vi "New Project.vi"(9 "DBSet":T1={"Server"="172.20.23.107", "DB"="HTPSDB", "PSW"="data'songyy", "User"="sa"}, 10 "UserID":string="L043460", 11 "厂区":string="清溪") -> ()   [LabVIEW 2011] (continued)
                            n505 = Index Array(array=w581) -> (element=w578:bool)  [unwired: 1 in]
                            n506 = local write "fre-save"(w574) -> ()
                            n507 = local write "AutoSN"(w578) -> ()
                          }
                          frame #2 {
                            n508 = disable-structure shown="禁用" {
                              disable-tunnel: w584 -> [w585 _]
                              frame Disabled {
                                n509 = local read "Luxshare_P/N:"() -> (w624:string)
                                n510 = local read "Luxshare_P/N:"() -> (w627:string)
                                n511 = local read "Luxshare_P/N:"() -> (w630:string)
                                n512 = local read "厂区"() -> ()  [unwired: 1 out]
                                n513 = local read "厂区"() -> (w586:string)
                                n514 = call "query.net.vi"() -> ()  [unwired: 10 in, 2 out]
                                n515 = call "_wmg_PNtoPNwhereConnect.vi"("Input"=w624) -> ("Output"=w598:string)
                                n516 = call "_wmg_PNtoPNwhereConnect.vi"("Input"=w630) -> ("Output"=w603:string)
                                n517 = call "_wmg_PNtoPNwhereConnect.vi"("Input"=w627) -> ("Output"=w601:string)
                                n518 = property on="System_Mode" class="Ring (严格)"() -> ("RingText.Text"=w597:string)  [unwired: 2 in, 2 out]
                                n519 = call "_wmg_HardModetoHardModewhereConnect.vi"("Input"=w597, "Factory"=w586) -> ("Output"=w588:string)
                                n520 = Concatenate Strings(w603, w588) -> (w602:string)
                                n521 = call "sql-readinfo_vproject.vi"("DBSet"=w585, "操作模式"=T7."查询数据", "查询项目"="Prjinf", "限定条件"=w602) -> ("ResultString"=w617:string)  [unwired: 13 in, 10 out]
                                n522 = local write "Project Information"(w617) -> ()
                                n523 = Concatenate Strings(w598, w588) -> (w596:string)
                                n524 = call "sql-readinfo_vproject.vi"("DBSet"=w585, "操作模式"=T7."查询数据", "查询项目"="SwitchMatrix", "限定条件"=w596) -> ("ResultString"=w619:string)  [unwired: 13 in, 10 out]
                                n525 = Concatenate Strings(w601, w588) -> (w600:string)
                                n526 = call "sql-readinfo_vproject.vi"("DBSet"=w585, "操作模式"=T7."查询数据", "查询项目"="Spec", "限定条件"=w600) -> ("ResultString"=→"Spec_midVar":string)  [unwired: 13 in, 10 out]
                                n527 = local write "Switch Matrix"(w619) -> ()
                                n528 = local read "Luxshare_P/N:"() -> (w609:string)
                                n529 = local read "Luxshare_P/N:"() -> (w612:string)
                                n530 = local read "Luxshare_P/N:"() -> (w615:string)
                                n531 = local read "Luxshare_P/N:"() -> (w621:string)
                                n532 = call "_wmg_PNtoPNwhereConnect.vi"("Input"=w609) -> ("Output"=w589:string)
                                n533 = Concatenate Strings(w589, w588) -> (w587:string)
                                n534 = call "_wmg_PNtoPNwhereConnect.vi"("Input"=w612) -> ("Output"=w591:string)
                                n535 = Concatenate Strings(w591, w588) -> (w590:string)
                                n536 = call "_wmg_PNtoPNwhereConnect.vi"("Input"=w615) -> ("Output"=w593:string)
                                n537 = Concatenate Strings(w593, w588) -> (w592:string)
                                n538 = call "sql-readinfo_vproject.vi"("DBSet"=w585, "操作模式"=T7."查询数据", "查询项目"="Spec_Points", "限定条件"=w587) -> ("ResultString"=w605:string)  [unwired: 13 in, 10 out]
                                n539 = call "sql-readinfo_vproject.vi"("DBSet"=w585, "操作模式"=T7."查询数据", "查询项目"="Switch_File_Path", "限定条件"=w592) -> ("ResultString"=w607:string)  [unwired: 13 in, 10 out]
                                n540 = call "_wmg_PNtoPNwhereConnect.vi"("Input"=w621) -> ("Output"=w595:string)
                                n541 = Concatenate Strings(w595, w588) -> (w594:string)
                                n542 = call "sql-readinfo_vproject.vi"("DBSet"=w585, "操作模式"=T7."查询数据", "查询项目"="LabelC", "限定条件"=w594) -> ("ResultString"=w618:string)  [unwired: 13 in, 10 out]
                                n543 = call "sql-readinfo_vproject.vi"("DBSet"=w585, "操作模式"=T7."查询数据", "查询项目"="Spec_File_Path", "限定条件"=w590) -> ("ResultString"=w606:string)  [unwired: 13 in, 10 out]
                                n544 = local write "Switch File Path"(w607) -> ()
                                n545 = Decimal String To Number(string=w605) -> (number=w604:i32)  [unwired: 2 in, 1 out]
                                n546 = local write "Spec Points"(w604) -> ()
                                n547 = local write "Spec File Path"(w606) -> ()
                                n548 = local write "Label Content"(w618) -> ()
                              }
                              frame Enabled {
                              }
                            }
                          }
                          frame #3 {
                            n549 = local read "Luxshare_P/N:"() -> (w647:string)
                            n550 = property on="System_Mode" class="Ring (严格)"() -> ("RingText.Text"=w646:string)  [unwired: 2 in, 2 out]
                            n551 = local read "厂区"() -> (w645:string)
                            n552 = Search and Replace String(input string="select SwitchMatrix ,Prjinf,Spec,LabelC,Switch_File_Path,Spec_File_Path,Spec_Points from vproject where LuxsharePN='@PN@' and HardWare_Mode='@Mode@' and  Factory ='@Facotry@'", search string="@PN@" ("搜索字符串"), replace string=w647) -> (result string=w651:string)  [unwired: 5 in, 3 out]
                            n553 = Search and Replace String(input string=w651, search string="@Mode@" ("搜索字符串"), replace string=w646) -> (result string=w649:string)  [unwired: 5 in, 3 out]
                            n554 = Search and Replace String(input string=w649, search string="@Facotry@" ("搜索字符串"), replace string=w645) -> (result string=w644:string)  [unwired: 5 in, 3 out]
                            n555 = call "query.net.vi"("Sql"=w644, "DBSet"=w643) -> ("result"=w642:string[][])  [unwired: 8 in, 1 out]
                            n556 = Index Array(array=w642, index (row)=0 ("索引 (行)")) -> (element=w640:string[])  [unwired: 1 in]
                            n557 = Index Array(array=w640) -> (element #1=w639:string, element #2=w638:string, element #3=w637:string, element #4=w636:string, element #5=w635:string, element #6=w634:string, element #7=w633:string)  [unwired: 7 in]
                            n558 = Decimal String To Number(string=w633) -> (number=w632:i32)  [unwired: 2 in, 1 out]
                            n559 = local write "Switch Matrix"(w639) -> ()
                            n560 = local write "Project Information"(w638) -> ()
                            n561 = local write "Switch File Path"(w635) -> ()
                            n562 = local write "Label Content"(w636) -> ()
                            n563 = local write "Spec_midVar"(w637) -> ()
                            n564 = local write "Spec File Path"(w634) -> ()
                            n565 = local write "Spec Points"(w632) -> ()
                          }
                          frame #4 {
                            n566 = local read "Spec_midVar"() -> (w655:string)
                            n567 = property on="Cable AWG:" class="Ring (严格)"() -> ("StringsAndValues[]"=w666:T10)  [unwired: 2 in, 2 out]
                            n568 = property on="Customer" class="Ring (严格)"() -> ("StringsAndValues[]"=w668:T10)  [unwired: 2 in, 2 out]
                            n569 = Search and Replace String(replace all?=TRUE ("替换全部？(F)"), input string=w655, search string="#" ("搜索字符串"), replace string="\t") -> (result string=w659:string)  [unwired: 4 in, 3 out]
                            n570 = local read "Customer"() -> (w667:string)
                            n571 = local read "AWG"() -> (w665:string)
                            n572 = Spreadsheet String To Array(format string="%s" ("格式字符串"), spreadsheet string=w659, array type (2D Dbl)=string[][] []) -> (array=w654:string[][])  [unwired: 1 in]
                            n573 = call "_wmg_downlistValue.vi"(1:"Customer"=w665, 2:"Customer"=w666) -> ("Customer"=w669:u16)
                            n574 = call "_wmg_downlistValue.vi"(1:"Customer"=w667, 2:"Customer"=w668) -> ("Customer"=w670:u16)
                            n575 = local write "Cable AWG:"(w669) -> ()
                            n576 = local write "Customer"(w670) -> ()
                            n577 = Array To Spreadsheet String(delimiter (Tab)="#" ("分隔符(Tab)"), array=w654, 3:"%s" ("格式字符串")) -> (spreadsheet string=w664:string)
                            n578 = local write "Spec String"(w664) -> ()
                            n579 = local write "Spec Associate"(w654) -> ()
                          }
                        }
                      }
                    }
                  }
                  frame #1 {
                    # "列数\n0. S-para Pair Name\n1. NEXT Pair Name\n2. FEXT Pair Name\n3. Diff TestItems\n4. Single TestItems\n5. TDR TestItems\n6. Spec Associate\n7. VNA Cal File Path\n8. Report Config\n9. ILD Spec\n10. TDR Setting"
                    # "解析Prjinf"
                    n580 = local read "Project Information"() -> (w705:string)
                    n581 = Spreadsheet String To Array(delimiter (Tab)="#" ("分隔符(Tab)"), format string="%s" ("格式字符串"), spreadsheet string=w705, array type (2D Dbl)=string[][] []) -> (array=w702:string[][])
                    n582 = Index Array(array=w702, index (col) #1=0 ("索引"), index (col) #2=1 ("索引 (列)"), index (col) #3=2 ("索引 (列)"), index (col) #4=3 ("索引 (列)"), index (col) #5=4 ("索引 (列)"), index (col) #6=5 ("索引"), index (col) #7=6 ("索引 (列)"), index (col) #8=7 ("索引 (列)"), index (col) #9=8 ("索引 (列)"), index (col) #10=9 ("索引 (列)"), index (col) #11=10 ("索引"), index (col) #12=11 ("索引 (列)"), index (col) #13=12 ("索引 (列)"), index (col) #14=13 ("索引 (列)"), index (col) #15=14 ("索引 (列)")) -> (element #1=w701:string[], element #2=w700:string[], element #3=w699:string[], element #4=w698:string[], element #5=w697:string[], element #6=w696:string[], element #7=w695:string[], element #8=w694:string[], element #9=w693:string[], element #10=w692:string[], element #11=w691:string[], element #12=w678:string[], element #13=w675:string[], element #14=w673:string[], element #15=w671:string[])  [unwired: 15 in]
                    n583 = stacked-sequence {
                      tunnel: w701 -> [_ w719 _ _ _ _ _ _ _]
                      tunnel: w700 -> [_ w718 _ _ _ _ _ _ _]
                      tunnel: w699 -> [_ w717 _ _ _ _ _ _ _]
                      tunnel: w698 -> [_ w716 _ _ _ _ _ _ _]
                      tunnel: w697 -> [_ w715 _ _ _ _ _ _ _]
                      tunnel: w696 -> [_ w714 _ _ _ _ _ _ _]
                      tunnel: w695 -> [_ _ w765 _ _ _ _ _ _]
                      tunnel: w694 -> [_ _ w764 _ _ _ _ _ _]
                      tunnel: w693 -> [_ _ _ w793 _ _ _ _ _]
                      tunnel: w692 -> [_ _ _ _ _ _ _ _ _]
                      tunnel: w691 -> [_ _ _ _ _ w813 _ _ _]
                      tunnel: w678 -> [_ _ _ _ _ _ w843 _ _]
                      tunnel: w675 -> [_ _ _ w785 _ _ _ _ _]
                      tunnel: w673 -> [_ _ _ _ _ _ _ w887 _]
                      tunnel: w671 -> [_ _ _ _ _ _ _ _ w894]
                      frame #0 {
                        n584 = local read "Single init"() -> (→"Single init 2":i32[])
                        n585 = local read "FEXT init"() -> (→"FEXT init 2":i32[])
                        n586 = local read "Diff init"() -> (→"Diff init 2":i32[])
                        n587 = local read "NEXT init"() -> (→"NEXT init 2":i32[])
                        n588 = local read "S-p init"() -> (→"S-p init 2":i32[])
                        n589 = local read "TDR init"() -> (→"TDR init 2":i32[])
                      }
                      frame #1 {
                        n590 = stacked-sequence {
                          tunnel: [_ w741 _ _] -> _
                          tunnel: w719 -> [_ w741 _ _]
                          tunnel: w718 -> [_ w734 _ _]
                          tunnel: w717 -> [_ _ w747 _]
                          tunnel: w716 -> [_ _ w742 _]
                          tunnel: w715 -> [_ _ _ w755]
                          tunnel: w714 -> [_ _ _ w752]
                          frame #0 {
                            n591 = local read "FEXT init"() -> (w727:string[])
                            n592 = local read "FEXT init"() -> (w726:i32[])
                            n593 = local read "NEXT init"() -> (w730:string[])
                            n594 = local read "NEXT init"() -> (w728:i32[])
                            n595 = local read "S-p init"() -> (w729:i32[])
                            n596 = local read "S-p init"() -> (w731:string[])
                            n597 = property on="S-para Pair Name" class="LstBox (严格)"("Item Names"=w731, "Item Symbols"=w729) -> ()  [unwired: 2 in, 2 out]
                            n598 = property on="NEXT Pair Name" class="LstBox (严格)"("Item Names"=w730, "Item Symbols"=w728) -> ()  [unwired: 2 in, 2 out]
                            n599 = property on="FEXT Pair Name" class="LstBox (严格)"("Item Names"=w727, "Item Symbols"=w726) -> ()  [unwired: 2 in, 2 out]
                            n600 = local read "Single init"() -> (w723:string[])
                            n601 = local read "Single init"() -> (w722:i32[])
                            n602 = local read "Diff init"() -> (w725:string[])
                            n603 = local read "Diff init"() -> (w724:i32[])
                            n604 = local read "TDR init"() -> (w721:string[])
                            n605 = local read "TDR init"() -> (w720:i32[])
                            n606 = property on="Diff Test Items" class="LstBox (严格)"("Item Names"=w725, "Item Symbols"=w724) -> ()  [unwired: 2 in, 2 out]
                            n607 = property on="Single Test Items" class="LstBox (严格)"("Item Names"=w723, "Item Symbols"=w722) -> ()  [unwired: 2 in, 2 out]
                            n608 = property on="TDR Test Items" class="LstBox (严格)"("Item Names"=w721, "Item Symbols"=w720) -> ()  [unwired: 2 in, 2 out]
                          }
                          frame #1 {
                            n609 = local read "S-p init"() -> (w739:i32[])
                            n610 = local read "S-p init"() -> (w733:string[])
                            n611 = local read "NEXT init"() -> (w732:string[])
                            n612 = local read "NEXT init"() -> (w735:i32[])
                            n613 = call "_wmg_readItems.vi"("input_p"=w739, "input"=w733, "input_sp"=w741) -> ("output_p"=w738:i32[], "output_sp"=w740:string[])
                            n614 = call "_wmg_readItems2.vi"("input_p"=w735, "input"=w732, "input_sp"=w734) -> ("output_p"=w736:i32[], "output_sp"=w737:string[])
                            n615 = property on="S-para Pair Name" class="LstBox (严格)"("Item Names"=w740, "Item Symbols"=w738) -> ()  [unwired: 2 in, 2 out]
                            n616 = property on="NEXT Pair Name" class="LstBox (严格)"("Item Names"=w737, "Item Symbols"=w736) -> ()  [unwired: 2 in, 2 out]
                          }
                          frame #2 {
                            n617 = local read "FEXT init"() -> (w750:string[])
                            n618 = local read "FEXT init"() -> (w751:i32[])
                            n619 = local read "Diff init"() -> (w746:string[])
                            n620 = local read "Diff init"() -> (w745:i32[])
                            n621 = call "_wmg_readItems2.vi"("input_p"=w745, "input"=w746, "input_sp"=w742) -> ("output_p"=w744:i32[], "output_sp"=w743:string[])
                            n622 = call "_wmg_readItems.vi"("input_p"=w751, "input"=w750, "input_sp"=w747) -> ("output_p"=w748:i32[], "output_sp"=w749:string[])
                            n623 = property on="FEXT Pair Name" class="LstBox (严格)"("Item Names"=w749, "Item Symbols"=w748) -> ()  [unwired: 2 in, 2 out]
                            n624 = property on="Diff Test Items" class="LstBox (严格)"("Item Names"=w743, "Item Symbols"=w744) -> ()  [unwired: 2 in, 2 out]
                          }
                          frame #3 {
                            n625 = local read "TDR init"() -> (w754:string[])
                            n626 = local read "TDR init"() -> (w753:i32[])
                            n627 = local read "Single init"() -> (w756:string[])
                            n628 = local read "Single init"() -> (w757:i32[])
                            n629 = call "_wmg_readItems.vi"("input_p"=w757, "input"=w756, "input_sp"=w755) -> ("output_p"=w759:i32[], "output_sp"=w758:string[])
                            n630 = call "_wmg_readItems2.vi"("input_p"=w753, "input"=w754, "input_sp"=w752) -> ("output_p"=w761:i32[], "output_sp"=w760:string[])
                            n631 = property on="TDR Test Items" class="LstBox (严格)"("Item Names"=w760, "Item Symbols"=w761) -> ()  [unwired: 2 in, 2 out]
                            n632 = property on="Single Test Items" class="LstBox (严格)"("Item Names"=w758, "Item Symbols"=w759) -> ()  [unwired: 2 in, 2 out]
                          }
                        }
                      }
                      frame #2 {
                        n633 = disable-structure shown="禁用" {
                          disable-tunnel: w765 -> [w766 _]
                          frame Disabled {
                            n634 = property on="Diff Test Items" class="LstBox (严格)"() -> ("Item Symbols"=w770:i32[], "Item Names"=w768:string[])  [unwired: 2 in, 2 out]
                            n635 = for {
                              tunnel: w770 -> [w776] mode=indexing
                              shift-right: [w771] -> w767
                              shift-left: string[] [] -> [w772]
                              tunnel: w768 -> [w773] mode=indexing
                              n636 = Not Equal?(x=w776, y=37) -> (x != y?=w774:bool)
                              n637 = case shown="假" w774 {
                                tunnel: w773 -> [_ w780]
                                tunnel: w772 -> [w777 w779]
                                tunnel: [w777 w778] -> w771
                                frame False {
                                }
                                frame True {
                                n638 = Insert Into Array(array=w779, new element=w780) -> (w778:string[])  [unwired: 1 in]
                                }
                              }
                            }
                            n639 = Build Array(w767, w766) -> ()  [unwired: 1 out]
                          }
                          frame Enabled {
                          }
                        }
                        n640 = Index Array(array=w764, index=0 ("索引")) -> (element=w763:string)
                        n641 = local write "VNA Cal File Path:"(w763) -> ()
                      }
                      frame #3 {
                        n642 = Index Array(array=w785, index=0 ("索引")) -> (element=w783:string)
                        n643 = Index Array(array=w793, index #1=0 ("索引"), index #3=2 ("索引")) -> (element #1=w790:string, element #2=w789:string, element #3=w787:string)  [unwired: 1 in]
                        n644 = Equal?(x=w783, y="TRUE") -> (x = y?=w781:bool)
                        n645 = String To Path(string=w790) -> (path=w791:path)
                        n646 = call "_wmg_ReportConfigDivided@.vi"("Input"=w789) -> ("Output"=w788:string[][])
                        n647 = call "_wmg_ReportConfigDivided@.vi"("Input"=w787) -> ("Output"=w786:string[][])
                        n648 = local write "Postion for Raw data"(w788) -> ()
                        n649 = local write "Postion for \"PN&Tester&Date\" etc Fields"(w786) -> ()
                        n650 = local write "Report Templete Path:"(w791) -> ()
                        n651 = local write "Cancel Dem2X?"(w781) -> ()
                      }
                      frame #4 {
                      }
                      frame #5 {
                        # "TDR Setting\n0. Start TimeNs\n1. Stop TimeNs\n2. Data Points\n3. Filter Risetime(ps)\n4. Compensation(ohm)\n5. Impedance Filter\n6. Impedance Spec:\n7. Delay Spec:\n8. skew Spec:\n9. IL 2X Data:"
                        n652 = Index Array(array=w813, index #1=0 ("索引"), index #2=1 ("索引"), index #3=2 ("索引"), index #4=3 ("索引"), index #5=4 ("索引"), index #6=5 ("索引"), index #7=6 ("索引"), index #8=9 ("索引"), index #9=8 ("索引")) -> (element #1=w805:string, element #2=w804:string, element #3=w803:string, element #4=w802:string, element #5=w801:string, element #6=w800:string, element #7=w799:string, element #8=w797:string, element #9=w795:string)
                        n653 = stacked-sequence {
                          tunnel: w805 -> [w840]
                          tunnel: w804 -> [w837]
                          tunnel: w803 -> [w835]
                          tunnel: w802 -> [w834]
                          tunnel: w801 -> [w831]
                          tunnel: w800 -> [w830]
                          tunnel: w799 -> [w827]
                          tunnel: w797 -> [w822]
                          tunnel: w795 -> [w816]
                          frame #0 {
                            n654 = call "_wmg_ImpSpecDivided@.vi"("Input"=w827) -> ("Output"=w826:string[][])
                            n655 = Spreadsheet String To Array(format string="%s" ("格式字符串"), spreadsheet string=w822, array type (2D Dbl)=dbl[] []) -> (array=w817:dbl[])  [unwired: 1 in]
                            n656 = Fract/Exp String To Number(string=w816) -> (number=w815:dbl)  [unwired: 3 in, 1 out]
                            n657 = local write "Skew max(ps)"(w815) -> ()
                            n658 = Insert Into Array(array=w826, index (col)=0 ("禁用的索引 (列)"), new element=string[] ["Mating Area", "Cable Area", "Cable End"]) -> (w824:string[][])  [unwired: 1 in]
                            n659 = local write "2X Thru  IL Data"(w817) -> ()
                            n660 = Decimal String To Number(string=w830) -> (number=w814:i32)  [unwired: 2 in, 1 out]
                            n661 = local write "Impedance Spec:"(w824) -> ()
                            n662 = Number To Boolean Array(number=w814) -> (Boolean array=w829:bool[])
                            n663 = Array To Spreadsheet String(array=w817, 3:"%s" ("格式字符串")) -> (spreadsheet string=w819:string)  [unwired: 1 in]
                            n664 = Fract/Exp String To Number(string=w831) -> (number=w832:dbl)  [unwired: 3 in, 1 out]
                            n665 = Index Array(array=w829) -> (element=w828:bool)  [unwired: 1 in]
                            n666 = Fract/Exp String To Number(string=w837) -> (number=w838:dbl)  [unwired: 3 in, 1 out]
                            n667 = Decimal String To Number(string=w835) -> (number=w836:i32)  [unwired: 2 in, 1 out]
                            n668 = Fract/Exp String To Number(string=w834) -> (number=w833:dbl)  [unwired: 3 in, 1 out]
                            n669 = local write "2X Thru String"(w819) -> ()
                            n670 = Fract/Exp String To Number(string=w840) -> (number=w839:dbl)  [unwired: 3 in, 1 out]
                            n671 = local write "Compensation(ohm)"(w832) -> ()
                            n672 = local write "Filter Risetime(ps)"(w833) -> ()
                            n673 = local write "Impedance Filter"(w828) -> ()
                            n674 = local write "Start TimeNs"(w839) -> ()
                            n675 = local write "StopTimeNs"(w838) -> ()
                            n676 = local write "Data Points"(w836) -> ()
                          }
                        }
                      }
                      frame #6 {
                        # "TDR Setting\n0. Start TimeNs\n1. Stop TimeNs\n2. Data Points\n3. Filter Risetime(ps)\n4. Compensation(ohm)\n5. Impedance Filter\n6. Impedance Spec:\n7. Delay Spec:\n8. skew Spec:\n9. IL 2X Data:"
                        n677 = Index Array(array=w843, index #1=0 ("索引"), index #2=1 ("索引"), index #3=2 ("索引"), index #4=3 ("索引"), index #5=4 ("索引"), index #6=5 ("索引"), index #7=6 ("索引"), index #8=9 ("索引"), index #9=8 ("索引")) -> (element #1=w852:string, element #2=w851:string, element #3=w850:string, element #4=w849:string, element #5=w848:string, element #6=w847:string, element #7=w846:string, element #8=w844:string, element #9=w841:string)
                        n678 = stacked-sequence {
                          tunnel: w852 -> [w883]
                          tunnel: w851 -> [w882]
                          tunnel: w850 -> [w881]
                          tunnel: w849 -> [w880]
                          tunnel: w848 -> [w879]
                          tunnel: w847 -> [w878]
                          tunnel: w846 -> [w876]
                          tunnel: w844 -> [w873]
                          tunnel: w841 -> [w863]
                          frame #0 {
                            (unwired) string[] ["Mating Area", "Cable Area"]
                            n679 = call "_wmg_ImpSpecDivided@.vi"("Input"=w876) -> ("Output"=w875:string[][])
                            n680 = Spreadsheet String To Array(format string="%s" ("格式字符串"), spreadsheet string=w873, array type (2D Dbl)=dbl[] []) -> ()  [unwired: 1 in, 1 out]
                            n681 = Fract/Exp String To Number(string=w863) -> (number=w862:dbl)  [unwired: 3 in, 1 out]
                            n682 = local write "Skew max(ps) 2"(w862) -> ()
                            n683 = Insert Into Array(array=w875, index (col)=0 ("禁用的索引 (列)"), new element=string[] ["Mating Area", "Cable Area", "Cable End"]) -> (w870:string[][])  [unwired: 1 in]
                            n684 = Decimal String To Number(string=w878) -> (number=w861:i32)  [unwired: 2 in, 1 out]
                            n685 = Number To Boolean Array(number=w861) -> (Boolean array=w877:bool[])
                            n686 = local write "Impedance Spec: 2"(w870) -> ()
                            n687 = Fract/Exp String To Number(string=w879) -> (number=w868:dbl)  [unwired: 3 in, 1 out]
                            n688 = Index Array(array=w877) -> (element=w869:bool)  [unwired: 1 in]
                            n689 = Fract/Exp String To Number(string=w882) -> (number=w865:dbl)  [unwired: 3 in, 1 out]
                            n690 = Decimal String To Number(string=w881) -> (number=w866:i32)  [unwired: 2 in, 1 out]
                            n691 = Fract/Exp String To Number(string=w880) -> (number=w867:dbl)  [unwired: 3 in, 1 out]
                            n692 = local write "Compensation(ohm) 2"(w868) -> ()
                            n693 = local write "Filter Risetime(ps) 2"(w867) -> ()
                            n694 = Fract/Exp String To Number(string=w883) -> (number=w864:dbl)  [unwired: 3 in, 1 out]
                            n695 = local write "Impedance Filter 2"(w869) -> ()
                            n696 = local write "Data Points 2"(w866) -> ()
                            n697 = local write "StopTimeNs 2"(w865) -> ()
                            n698 = local write "Start TimeNs 2"(w864) -> ()
                          }
                        }
                      }
                      frame #7 {
                        n699 = Index Array(array=w887, index=0 ("索引")) -> (element=w885:string)
                        n700 = Decimal String To Number(string=w885) -> (number=w884:i32)  [unwired: 2 in, 1 out]
                        n701 = local write "平滑点数"(w884) -> ()
                      }
                      frame #8 {
                        n702 = Index Array(array=w894, index=0 ("索引")) -> (element=w892:string)
                        n703 = call "_wmg_ImpSpecDivided@.vi"("Input"=w892) -> ("Output"=w891:string[][])
                        n704 = Insert Into Array(array=w891, index (col)=0 ("禁用的索引 (列)"), new element=string[] ["Mating Area", "Cable Area", "Cable End"]) -> (w888:string[][])  [unwired: 1 in]
                        n705 = local write "Common Impedance Spec"(w888) -> ()
                      }
                    }
                    n706 = disable-structure shown="禁用" {
                      frame Disabled {
                        n707 = local read "2X Thru  IL Data"() -> ()  [unwired: 1 in]
                        n708 = Array To Spreadsheet String(3:"%s" ("格式字符串")) -> (spreadsheet string=w706:string)  [unwired: 2 in]
                        n709 = local write "2X Thru String"(w706) -> ()
                      }
                      frame Enabled {
                      }
                    }
                  }
                  frame #2 {
                    w903 = T4 {"Row"=0, "Column"=0} ("编辑位置")
                    w904 = u32 4 ("列数")
                    n710 = property on="Single Test Items" class="LstBox (严格)"() -> ("Item Names"=w911:string[], "Item Symbols"=w910:i32[])  [unwired: 2 in, 2 out]
                    n711 = property on="TDR Test Items" class="LstBox (严格)"() -> ("Item Names"=w909:string[], "Item Symbols"=w908:i32[])  [unwired: 2 in, 2 out]
                    n712 = property on="Diff Test Items" class="LstBox (严格)"() -> ("Item Names"=w913:string[], "Item Symbols"=w912:i32[])  [unwired: 2 in, 2 out]
                    n713 = call "_wmg_SelectItems2.vi"("Item Syms"=w908, "Item name"=w909) -> ("Selected tem"=w907:string[])  [unwired: 7 in, 2 out]
                    n714 = call "_wmg_SelectItems2.vi"("Item Syms"=w912, "Item name"=w913) -> ("Selected tem"=w906:string[])  [unwired: 7 in, 2 out]
                    n715 = call "_wmg_SelectItems2.vi"("Item Syms"=w910, "Item name"=w911) -> ("Selected tem"=w905:string[])  [unwired: 7 in, 2 out]
                    n716 = property on="Postion for Raw data" class="Tbl (严格)"() -> ("Value"=w902:string[][])  [unwired: 2 in, 2 out]
                    n717 = Insert Into Array(array=w907, new element #1=w906, new element #2=w905) -> (w901:string[])  [unwired: 1 in]
                    n718 = local read "2X Thru  IL Data"() -> (w897:dbl[])
                    n719 = Replace Array Subset(array=w902, new element=w901, index (col)=0 ("禁用的索引 (列)")) -> (w900:string[][])  [unwired: 1 in]
                    n720 = property on="Postion for Raw data" class="Tbl (严格)"("Value"=w900) -> ()  [unwired: 2 in, 2 out]
                    n721 = Array Size(array=w897) -> (size(s)=w896:i32)
                    n722 = for {
                      N: w896 -> [_]
                      tunnel: [w914] -> w895 mode=indexing
                      i -> [w914]
                    }
                    n723 = Bundle(w895, "2X Thru  IL Data"=w897) -> (w898:cluster{i32[], "2X Thru  IL Data":dbl[]})  [unwired: 1 in]
                    n724 = local write "Insertion Loss"(w898) -> ()
                    n725 = property on="Postion for Raw data" class="Tbl (严格)"("Number of Columns"=w904, "EditPos"=w903) -> ()  [unwired: 2 in, 2 out]
                    n726 = property on="Postion for \"PN&Tester&Date\" etc Fields" class="Tbl (严格)"("Number of Columns"=w904, "EditPos"=w903) -> ()  [unwired: 2 in, 2 out]
                  }
                  frame #3 {
                    n727 = local read "Local"() -> (w915:bool)
                    n728 = case shown="真" w915 {
                      frame False {
                        n729 = local read "result_query"() -> (w919:string)
                        n730 = call <vilib>:"Trim Whitespace.vi"("string"=w919) -> ("trimmed string"=w918:string)  [unwired: 1 in]
                        n731 = String Length(string=w918) -> (length=w917:i32)
                        n732 = Equal To 0?(x=w917) -> (x = 0?=w916:bool)
                        n733 = case shown="假" w916 {
                          frame False {
                            n734 = property on="Update" class="Bool (严格)"("DisabledEnum"=T5."Enabled" ("禁用")) -> ()  [unwired: 2 in, 2 out]
                            n735 = property on="Delete" class="Bool (严格)"("DisabledEnum"=T5."Enabled" ("禁用")) -> ()  [unwired: 2 in, 2 out]
                          }
                          frame True {
                            n736 = local write "Luxshare_P/N:"("") -> ()
                            n737 = One Button Dialog(message="数据库中无此记录" ("消息")) -> ()  [unwired: 1 in, 1 out]
                          }
                        }
                      }
                      frame True {
                        n738 = local read "fileexist"() -> (w925:bool)
                        n739 = Not(x=w925) -> (.not. x?=w924:bool)
                        n740 = case shown="假" w924 {
                          frame False {
                            # "文件不存在"
                            n741 = local read "Impedance Spec:"() -> (w929:string[][])
                            n742 = local write "Luxshare_P/N:"("") -> ()
                            n743 = Replace Array Subset(array=w929, new element=string[] ["", "", ""] ("新元素/子数组"), index (col)=0 ("禁用的索引 (列)")) -> (w928:string[][])  [unwired: 1 in]
                            n744 = local write "Impedance Spec:"(w928) -> ()
                            n745 = property on="Update" class="Bool (严格)"("DisabledEnum"=T5."Disabled and Grayed Out" ("禁用")) -> ()  [unwired: 2 in, 2 out]
                            n746 = property on="Delete" class="Bool (严格)"("DisabledEnum"=T5."Disabled and Grayed Out" ("禁用")) -> ()  [unwired: 2 in, 2 out]
                          }
                          frame True {
                            n747 = property on="Update" class="Bool (严格)"("DisabledEnum"=T5."Enabled" ("禁用")) -> ()  [unwired: 2 in, 2 out]
                            n748 = property on="Delete" class="Bool (严格)"("DisabledEnum"=T5."Enabled" ("禁用")) -> ()  [unwired: 2 in, 2 out]
                          }
                        }
                      }
                    }
                  }
                }
              }
              frame 100 {
                n749 = stacked-sequence {
                  tunnel: w935 -> [w936 w955 _]
                  frame #0 {
                    n750 = local read "Local"() -> (w937:bool)
                    n751 = case shown="真" w937 {
                      tunnel: w936 -> [w948 _]
                      frame False {
                        n752 = local read "Luxshare_P/N:"() -> (w940:string)
                        n753 = Search and Replace String(input string="delete from vproject where LuxsharePN='@PN@' and HardWare_Mode='@Mode@' and  Factory ='@Facotry@'", search string="@PN@" ("搜索字符串"), replace string=w940) -> (result string=w946:string)  [unwired: 5 in, 3 out]
                        n754 = property on="System_Mode" class="Ring (严格)"() -> ("RingText.Text"=w939:string)  [unwired: 2 in, 2 out]
                        n755 = Search and Replace String(input string=w946, search string="@Mode@" ("搜索字符串"), replace string=w939) -> (result string=w944:string)  [unwired: 5 in, 3 out]
                        n756 = local read "厂区"() -> (w938:string)
                        n757 = Search and Replace String(input string=w944, search string="@Facotry@" ("搜索字符串"), replace string=w938) -> (result string=w941:string)  [unwired: 5 in, 3 out]
                        n758 = call "query.net.vi"("Sql"=w941, "DBSet"=w948) -> ()  [unwired: 8 in, 2 out]
                      }
                      frame True {
                        n759 = local read "Luxshare_P/N:"() -> (w950:string)
                        n760 = call <vilib>:"Application Directory.vi"() -> ("Application Directory"=w954:path)
                        n761 = Concatenate Strings("Database\\" ("字符串"), w950, ".hpj" ("字符串")) -> (w953:string)
                        n762 = Build Path(base path=w954, name or relative path=w953) -> (appended path=w949:path)
                        n763 = Delete(path (use dialog)=w949) -> ()  [unwired: 4 in, 3 out]
                      }
                    }
                  }
                  frame #1 {
                    n764 = stacked-sequence {
                      tunnel: w955 -> [_ _ _ _ w1139 _]
                      frame #0 {
                        w985 = "@"
                        w986 = "\r\n"
                        w995 = "%s" ("格式字符串")
                        n765 = local read "Impedance Filter"() -> (w972:bool)
                        n766 = local read "Impedance Spec:"() -> (w997:string[][])
                        n767 = local read "2X Thru String"() -> (w982:string)
                        n768 = property on="Skew max(ps)" class="DigNum (严格)"() -> ("NumText.Text"=w974:string)  [unwired: 2 in, 2 out]
                        n769 = property on="Delay(ns)" class="DigNum (严格)"() -> ("NumText.Text"=w981:string)  [unwired: 2 in, 2 out]
                        n770 = property on="Start TimeNs" class="DigNum (严格)"() -> ("NumText.Text"=w980:string)  [unwired: 2 in, 2 out]
                        n771 = property on="StopTimeNs" class="DigNum (严格)"() -> ("NumText.Text"=w979:string)  [unwired: 2 in, 2 out]
                        n772 = property on="Data Points" class="DigNum (严格)"() -> ("NumText.Text"=w978:string)  [unwired: 2 in, 2 out]
                        n773 = property on="Filter Risetime(ps)" class="DigNum (严格)"() -> ("NumText.Text"=w977:string)  [unwired: 2 in, 2 out]
                        n774 = property on="Compensation(ohm)" class="DigNum (严格)"() -> ("NumText.Text"=w976:string)  [unwired: 2 in, 2 out]
                        n775 = Boolean To (0,1)(Boolean=w972) -> (0, 1=w999:i16)
                        n776 = Number To Decimal String(number=w999) -> (decimal integer string=w998:string)  [unwired: 1 in]
                        n777 = call "impedance spec.vi"("Impedance Spec:"=w997) -> ("Impedance spec string"=w996:string)  [unwired: 10 in]
                        n778 = call <vilib>:"Trim Whitespace.vi"("string"=w982) -> ("trimmed string"=w971:string)  [unwired: 1 in]
                        n779 = Build Array(w980, w979, w978, w977, w976, w998, w996, w981, w974, w971) -> (w975:string[])
                        n780 = local read "2X Thru String"() -> (w969:string)
                        n781 = local read "Report Templete Path:"() -> (w983:path)
                        n782 = property on="Postion for Raw data" class="Tbl (严格)"() -> ("Value"=w994:string[][])  [unwired: 2 in, 2 out]
                        n783 = local write "TDR Setting"(w975) -> ()
                        n784 = property on="Postion for \"PN&Tester&Date\" etc Fields" class="Tbl (严格)"() -> ("Value"=w993:string[][])  [unwired: 2 in, 2 out]
                        n785 = local read "Impedance Filter 2"() -> (w956:bool)
                        n786 = Array To Spreadsheet String(array=w994, 3:w995) -> (spreadsheet string=w991:string)  [unwired: 1 in]
                        n787 = Array To Spreadsheet String(array=w993, 3:w995) -> (spreadsheet string=w989:string)  [unwired: 1 in]
                        n788 = local read "Impedance Spec: 2"() -> (w962:string[][])
                        n789 = Path To String(path=w983) -> (string=w984:string)
                        n790 = property on="Delay(ns)" class="DigNum (严格)"() -> ("NumText.Text"=w960:string)  [unwired: 2 in, 2 out]
                        n791 = property on="Skew max(ps) 2" class="DigNum (严格)"() -> ("NumText.Text"=w959:string)  [unwired: 2 in, 2 out]
                        n792 = property on="Start TimeNs 2" class="DigNum (严格)"() -> ("NumText.Text"=w968:string)  [unwired: 2 in, 2 out]
                        n793 = property on="StopTimeNs 2" class="DigNum (严格)"() -> ("NumText.Text"=w967:string)  [unwired: 2 in, 2 out]
                        n794 = property on="Data Points 2" class="DigNum (严格)"() -> ("NumText.Text"=w966:string)  [unwired: 2 in, 2 out]
                        n795 = property on="Filter Risetime(ps) 2" class="DigNum (严格)"() -> ("NumText.Text"=w965:string)  [unwired: 2 in, 2 out]
                        n796 = property on="Compensation(ohm) 2" class="DigNum (严格)"() -> ("NumText.Text"=w964:string)  [unwired: 2 in, 2 out]
                        n797 = Search and Replace String(replace all?=TRUE ("替换全部？(F)"), input string=w991, search string=w986, replace string=w985) -> (result string=w988:string)  [unwired: 4 in, 3 out]
                        n798 = Search and Replace String(replace all?=TRUE ("替换全部？(F)"), input string=w989, search string=w986, replace string=w985) -> (result string=w987:string)  [unwired: 4 in, 3 out]
                        n799 = Boolean To (0,1)(Boolean=w956) -> (0, 1=w970:i16)
                        n800 = Build Array(w984, w988, w987) -> (w973:string[])
                        n801 = Number To Decimal String(number=w970) -> (decimal integer string=w963:string)  [unwired: 1 in]
                        n802 = call "impedance spec.vi"("Impedance Spec:"=w962) -> ("Impedance spec string"=w961:string)  [unwired: 10 in]
                        n803 = call <vilib>:"Trim Whitespace.vi"("string"=w969) -> ("trimmed string"=w958:string)  [unwired: 1 in]
                        n804 = local write "Report Config"(w973) -> ()
                        n805 = Build Array(w968, w967, w966, w965, w964, w963, w961, w960, w959, w958) -> (w957:string[])
                        n806 = local write "TDR Setting2"(w957) -> ()
                      }
                      frame #1 {
                        n807 = local read "Common Impedance Spec"() -> (w1003:string[][])
                        n808 = property on="S-para Pair Name" class="LstBox (严格)"() -> ("Item Names"=w1038:string[], "Item Symbols"=w1037:i32[])  [unwired: 2 in, 2 out]
                        n809 = property on="NEXT Pair Name" class="LstBox (严格)"() -> ("Item Names"=w1036:string[], "Item Symbols"=w1035:i32[])  [unwired: 2 in, 2 out]
                        n810 = property on="FEXT Pair Name" class="LstBox (严格)"() -> ("Item Names"=w1034:string[], "Item Symbols"=w1033:i32[])  [unwired: 2 in, 2 out]
                        n811 = property on="Single Test Items" class="LstBox (严格)"() -> ("Item Names"=w1040:string[], "Item Symbols"=w1039:i32[])  [unwired: 2 in, 2 out]
                        n812 = property on="Diff Test Items" class="LstBox (严格)"() -> ("Item Names"=w1042:string[], "Item Symbols"=w1041:i32[])  [unwired: 2 in, 2 out]
                        n813 = property on="TDR Test Items" class="LstBox (严格)"() -> ("Item Names"=w1020:string[], "Item Symbols"=w1019:i32[])  [unwired: 2 in, 2 out]
                        n814 = call "impedance spec.vi"("Impedance Spec:"=w1003) -> ("Impedance spec string"=w1002:string)  [unwired: 10 in]
                        n815 = call "Selected items.vi"("Item Syms"=w1037, "Item name"=w1038) -> ("Selected tem"=w1032:string[])  [unwired: 7 in, 2 out]
                        n816 = call "Selected items.vi"("Item Syms"=w1035, "Item name"=w1036) -> ("Selected tem"=w1031:string[])  [unwired: 7 in, 2 out]
                        n817 = call "Selected items.vi"("Item Syms"=w1033, "Item name"=w1034) -> ("Selected tem"=w1030:string[])  [unwired: 7 in, 2 out]
                        n818 = call "Selected items.vi"("Item Syms"=w1041, "Item name"=w1042) -> ("Selected tem"=w1029:string[])  [unwired: 7 in, 2 out]
                        n819 = call "Selected items.vi"("Item Syms"=w1039, "Item name"=w1040) -> ("Selected tem"=w1028:string[])  [unwired: 7 in, 2 out]
                        n820 = call "Selected items.vi"("Item Syms"=w1019, "Item name"=w1020) -> ("Selected tem"=w1018:string[])  [unwired: 7 in, 2 out]
                        n821 = Build Array(w1002) -> (w1001:string[])
                        n822 = local read "VNA Cal File Path:"() -> (w1015:string)
                        n823 = local read "ILD Spec"() -> (w1014:u16)
                        n824 = local read "Report Config"() -> (w1016:string[])
                        n825 = local read "TDR Setting2"() -> (w1012:string[])
                        n826 = local read "Cancel Dem2X?"() -> (w1011:bool)
                        n827 = local read "TDR Setting"() -> (w1017:string[])
                        n828 = Number To Decimal String(number=w1014) -> (decimal integer string=w1022:string)  [unwired: 1 in]
                        n829 = Build Array(w1015) -> (w1027:string[])
                        n830 = Build Array(w1022) -> (w1021:string[])
                        n831 = Number To Decimal String(number="平滑点数") -> (decimal integer string=w1005:string)  [unwired: 1 in]
                        n832 = Select(t="TRUE", s=w1011, f="FALSE") -> (s? t:f=w1008:string)
                        n833 = Build Array(w1005) -> (w1004:string[])
                        n834 = Build Array(w1008) -> (w1007:string[])
                        n835 = Build Array(w1032, w1031, w1030, w1029, w1028, w1018, string[] ["占位符"], w1027, w1016, w1021, w1017, w1012, w1007, w1004, w1001) -> (w1026:string[][])
                        n836 = Transpose 2D Array(2D array=w1026) -> (transposed array=w1025:string[][])
                        n837 = Array To Spreadsheet String(delimiter (Tab)="#" ("分隔符(Tab)"), array=w1025, 3:"%s" ("格式字符串")) -> (spreadsheet string=w1013:string)
                        n838 = local write "Project Information"(w1013) -> ()
                      }
                      frame #2 {
                        n839 = local read "VNA Cal File Path:"() -> (w1062:string)
                        n840 = property on="Diff Test Items" class="LstBox (严格)"() -> ("Item Symbols"=w1059:i32[])  [unwired: 2 in, 2 out]
                        n841 = property on="Single Test Items" class="LstBox (严格)"() -> ("Item Symbols"=w1058:i32[])  [unwired: 2 in, 2 out]
                        n842 = property on="TDR Test Items" class="LstBox (严格)"() -> ("Item Symbols"=w1057:i32[])  [unwired: 2 in, 2 out]
                        n843 = property on="S-para Pair Name" class="LstBox (严格)"() -> ("Item Symbols"=w1056:i32[])  [unwired: 2 in, 2 out]
                        n844 = property on="NEXT Pair Name" class="LstBox (严格)"() -> ("Item Symbols"=w1055:i32[])  [unwired: 2 in, 2 out]
                        n845 = property on="FEXT Pair Name" class="LstBox (严格)"() -> ("Item Symbols"=w1051:i32[])  [unwired: 2 in, 2 out]
                        n846 = local read "Luxshare_P/N:"() -> (w1049:string)
                        n847 = local read "Length(mm):"() -> (w1063:string)
                        n848 = String Length(string=w1049) -> (length=w1050:i32)
                        n849 = Empty String/Path?(string/path=w1062) -> (empty?=w1060:bool)
                        n850 = Empty String/Path?(string/path=w1063) -> (empty?=w1061:bool)
                        n851 = Build Array(w1059, w1058, w1057, w1056, w1055, w1051) -> (w1054:i32[][])
                        n852 = Not(x=w1061) -> (.not. x?=w1053:bool)
                        n853 = Not(x=w1060) -> (.not. x?=w1052:bool)
                        n854 = Greater Than 0?(x=w1050) -> (x > 0?=w1048:bool)
                        n855 = call "_wmg_whetherItemsEmpty.vi"("Input"=w1054) -> ("bool"=w1064:bool)
                        n856 = local read "Spec Associate"() -> (w1043:string[][])
                        n857 = Compound Arithmetic op=AND(w1048, w1053, w1052, w1064) -> (w1047:bool)
                        n858 = local write "save?"(w1047) -> ()
                        n859 = Array To Spreadsheet String(delimiter (Tab)="#" ("分隔符(Tab)"), array=w1043, 3:"%s" ("格式字符串")) -> (spreadsheet string=w1046:string)
                        n860 = local write "Spec String"(w1046) -> ()
                      }
                      frame #3 {
                        n861 = local read "Local"() -> (w1065:bool)
                        n862 = case shown="假" w1065 {
                          frame False {
                            # "17"
                            # "16"
                            # "15"
                            # "14"
                            # "13"
                            # "11"
                            # "10"
                            # "9"
                            # "8"
                            # "7"
                            # "6"
                            # "5"
                            # "4"
                            # "3"
                            # "2"
                            # "1"
                            n863 = Format Date/Time String(time format string (%c)="%Y-%m-%d : %H:%M" ("时间格式字符串(%c)")) -> (date/time string=w1066:string)  [unwired: 2 in]
                            n864 = local read "Label Print?"() -> (w1077:bool)
                            n865 = local read "fre-save"() -> (w1084:string[])
                            n866 = local read "UserID"() -> (w1069:string)
                            n867 = Boolean To (0,1)(Boolean=w1077) -> (0, 1=w1102:i16)
                            n868 = local read "EEPROM Write/Read ?"() -> (w1078:bool)
                            n869 = local read "Sample Description:"() -> (w1098:string)
                            n870 = local read "Project Information"() -> (w1099:string)
                            n871 = Array To Spreadsheet String(delimiter (Tab)="," ("分隔符(Tab)"), array=w1084, 3:"" ("格式字符串")) -> (spreadsheet string=w1081:string)
                            n872 = local read "厂区"() -> (w1071:string)
                            n873 = Number To Decimal String(number=w1102) -> (decimal integer string=w1092:string)  [unwired: 1 in]
                            n874 = Concatenate Strings(w1069, " updated@ " ("字符串"), w1066) -> (w1068:string)
                            n875 = local read "Customer_P/N:"() -> (w1101:string)
                            n876 = local read "Switch File Path"() -> (w1076:string)
                            n877 = local read "Switch Matrix"() -> (w1094:string)
                            n878 = local read "Label Content"() -> (w1091:string)
                            n879 = local read "Length(mm):"() -> (w1096:string)
                            n880 = local read "Spec String"() -> (w1095:string)
                            n881 = call <vilib>:"Trim Whitespace.vi"("string"=w1081) -> ("trimmed string"=w1080:string)  [unwired: 1 in]
                            n882 = property on="Customer" class="Ring (严格)"() -> ("RingText.Text"=w1100:string)  [unwired: 2 in, 2 out]
                            n883 = property on="Cable AWG:" class="Ring (严格)"() -> ("RingText.Text"=w1097:string)  [unwired: 2 in, 2 out]
                            n884 = local read "FixtureNo"() -> (w1089:string)
                            n885 = local read "Label Num"() -> (w1104:string)
                            n886 = local read "Remark:"() -> (w1090:string)
                            n887 = Boolean To (0,1)(Boolean=w1078) -> (0, 1=w1103:i16)
                            n888 = local read "AutoSN"() -> (w1086:bool)
                            n889 = Number To Decimal String(number=w1103) -> (decimal integer string=w1093:string)  [unwired: 1 in]
                            n890 = Boolean To (0,1)(Boolean=w1086) -> (0, 1=w1087:i16)
                            n891 = Number To Decimal String(number=w1087) -> (decimal integer string=w1085:string)  [unwired: 1 in]
                            n892 = local read "Luxshare_P/N:"() -> (w1088:string)
                            n893 = local read "Spec File Path"() -> (w1075:string)
                            n894 = local read "Spec Points"() -> (w1074:dbl)
                            n895 = property on="System_Mode" class="Ring (严格)"() -> ("RingText.Text"=w1072:string)  [unwired: 2 in, 2 out]
                            n896 = Number To Decimal String(number=w1074) -> (decimal integer string=w1073:string)  [unwired: 1 in]
                            n897 = Build Array(w1088, w1101, w1100, w1099, w1098, w1097, w1096, w1095, w1094, w1093, w1089, w1092, w1104, w1091, w1090, w1085, w1080, w1076, w1075, w1073, w1072, w1071, w1068) -> (w1079:string[])
                            n898 = local write "Project File"(w1079) -> ()
                          }
                          frame True {
                            # "20"
                            # "19"
                            # "11"
                            # "10"
                            # "9"
                            # "8"
                            # "7"
                            # "6"
                            # "5"
                            # "4"
                            # "3"
                            # "2"
                            # "1"
                            n899 = local read "Label Print?"() -> (w1111:bool)
                            n900 = local read "fre-save"() -> (w1118:string[])
                            n901 = Boolean To (0,1)(Boolean=w1111) -> (0, 1=w1136:i16)
                            n902 = local read "EEPROM Write/Read ?"() -> (w1113:bool)
                            n903 = local read "Sample Description:"() -> (w1132:string)
                            n904 = local read "Project Information"() -> (w1133:string)
                            n905 = Array To Spreadsheet String(delimiter (Tab)="," ("分隔符(Tab)"), array=w1118, 3:"" ("格式字符串")) -> (spreadsheet string=w1115:string)
                            n906 = local read "SNType"() -> (w1112:string)
                            n907 = Number To Decimal String(number=w1136) -> (decimal integer string=w1126:string)  [unwired: 1 in]
                            n908 = local read "Customer_P/N:"() -> (w1135:string)
                            n909 = local read "Switch Matrix"() -> (w1128:string)
                            n910 = local read "Label Content"() -> (w1125:string)
                            n911 = local read "Length(mm):"() -> (w1130:string)
                            n912 = local read "Spec String"() -> (w1129:string)
                            n913 = property on="CmdType" class="Ring (严格)"() -> ("RingText.Text"=w1110:string)  [unwired: 2 in, 2 out]
                            n914 = call <vilib>:"Trim Whitespace.vi"("string"=w1115) -> ("trimmed string"=w1107:string)  [unwired: 1 in]
                            n915 = property on="Customer" class="Ring (严格)"() -> ("RingText.Text"=w1134:string)  [unwired: 2 in, 2 out]
                            n916 = property on="Cable AWG:" class="Ring (严格)"() -> ("RingText.Text"=w1131:string)  [unwired: 2 in, 2 out]
                            n917 = local read "FixtureNo"() -> (w1123:string)
                            n918 = local read "Label Num"() -> (w1138:string)
                            n919 = local read "Remark:"() -> (w1124:string)
                            n920 = local read "Switch File Path"() -> (w1108:string)
                            n921 = Boolean To (0,1)(Boolean=w1113) -> (0, 1=w1137:i16)
                            n922 = local read "AutoSN"() -> (w1120:bool)
                            n923 = Number To Decimal String(number=w1137) -> (decimal integer string=w1127:string)  [unwired: 1 in]
                            n924 = Boolean To (0,1)(Boolean=w1120) -> (0, 1=w1121:i16)
                            n925 = Number To Decimal String(number=w1121) -> (decimal integer string=w1119:string)  [unwired: 1 in]
                            n926 = local read "Luxshare_P/N:"() -> (w1122:string)
                            n927 = local read "Spec File Path"() -> (w1109:string)
                            n928 = local read "Spec Points"() -> (w1106:dbl)
                            n929 = Number To Decimal String(number=w1106) -> (decimal integer string=w1105:string)  [unwired: 1 in]
